vi "Read Enabled Channels.vi"(8 "error in (no error)":errorcluster, 11 "Time Parser in":refnum<class "Time Parser.lvclass">) -> (0 "error out":errorcluster, 2 "Enabled Channels":string[](array[string]), 3 "Time Parser out":refnum<class "Time Parser.lvclass">)   [LabVIEW 2015, in "Time Parser.lvclass"]
doc: "Time Parser.lvclass:Read Enabled Channels.vi\n\nThis VI returns the list of channel names that are enabled for the Time Parser class..\n\nInstrument Communication Module Version 1.0\nSeptember, 2017 Original Code Consulting David Thomson\n www.originalcode.com"
uses:
  Time Parser.lvclass
  Time Parser.lvclass/Time Parser.ctl
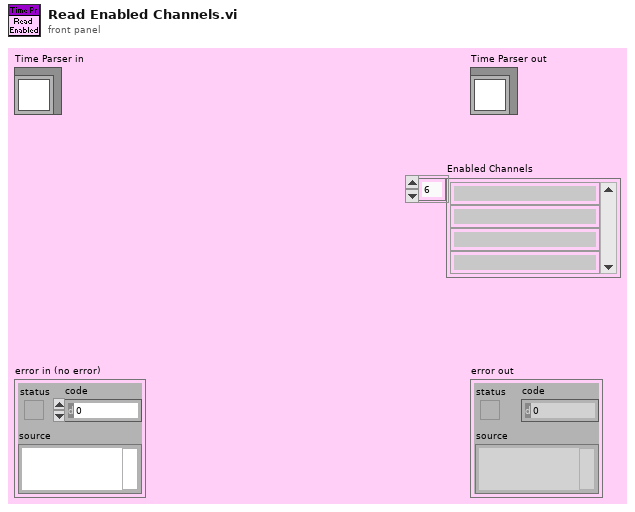
[diagram p1: front panel]
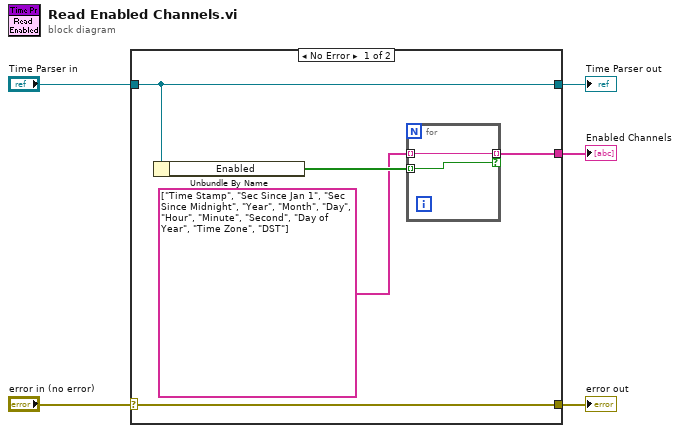
[diagram p0: block diagram]
diagram:
  n1 = case shown="No Error" "error in (no error)" {
    selector: "error in (no error)" -> [w10 w13]
    tunnel: [w10 w13] -> w4
    tunnel: [w9 w14] -> w2
    tunnel: "Time Parser in" -> [w9 w14]
    tunnel: [w8 _] -> w1
    frame No Error {
      n2 = Unbundle By Name(w9) -> ("Enabled"=w7:bool[])
      n3 = for {
        tunnel: [w12] -> w8 mode=indexing if=w11
        tunnel: string[] ["Time Stamp", "Sec Since Jan 1", "Sec Since Midnight", "Year", "Month", "Day", "Hour", "Minute", "Second", "Day of Year", "Time Zone", "DST"] -> [w12] mode=indexing
        tunnel: w7 -> [w11] mode=indexing
      }
    }
    frame Error {
    }
  }
  "error out" <- w4
  "Time Parser out" <- w2
  "Enabled Channels" <- w1
